vi "Barcode 2D_Setting_UI.vi"(6 "Analysis_Setting In":T2={"PreProcess"=enum."*Algorithm*", "Parameter"=""}, 8 "error in (no error)":errorcluster, 9 "ProjectName":string, 10 "ROI List IN":refnum<vi>, 11 "Vision_Image":T20(plugin-control)) -> (0 "error out":errorcluster, 1 "Cancel?":bool, 3 "Analysis_Setting":T2={"PreProcess"=enum."*Algorithm*", "Parameter"=""})   [LabVIEW 2019]
uses:
  <vilib>/vision/Instrument.llb/Demodulation Mode.ctl
  <vilib>/vision/Instrument.llb/Cell Sample Size.ctl
  <vilib>/vision/Instrument.llb/Cell Filter Mode.ctl
  <vilib>/vision/Instrument.llb/QR Code Search Options.ctl
  <vilib>/vision/Instrument.llb/Data Matrix Polarity.ctl
  <vilib>/vision/Instrument.llb/QR Code Model Type.ctl
  <vilib>/vision/Instrument.llb/QR Code Description Options.ctl
  Controls/_UI Command Cluster/Barcode 2D_UI Command Cluster.ctl
  Controls/Analysis_Type.ctl
  Controls/Analysis_Setting.ctl
  Controls/Barcode 2D/Analysis_Barcode 2D_Parameter.ctl
  <vilib>/vision/Instrument.llb/Data Matrix Search Options.ctl
  <vilib>/vision/Instrument.llb/Data Matrix Mirror.ctl
  <vilib>/vision/Instrument.llb/Cell Fill Percentage.ctl
  <vilib>/vision/Instrument.llb/ECC Type.ctl
  <vilib>/vision/Instrument.llb/Data Matrix Description Options.ctl
  <vilib>/vision/Instrument.llb/Data Matrix Advanced Options.ctl
  <vilib>/vision/Instrument.llb/Data Matrix Size Options.ctl
  Controls/V_Analysis_Type.ctl
  Ctrl/VisionProcessName.ctl
panel:
  in  "ROI":T1
  in  "Done":bool
  in  "Cancel":bool
  in  "ClampTab":T4(tab)
  in  "Suggest":bool
  in  "Barcode Type":enum16{"Data Matrix", "PDF417", "QR Code"}(ring)
  in  "Data Matrix Description Options":T5={"Aspect Ratio"=0.0, "Rows"=0, "Columns"=0, "Rectangle"=FALSE, "ECC"=-2, "Barcode Polarity"=-2, "Cell Fill Percentage"=-2, "Minimum Border Integrity %"=80.0, "Mirror Mode"=-2} {"Mirror Mode" items=["Auto-detect"=-2, "Normal"=0, "Mirrored"=1]; "ECC" items=["Auto-detect"=-2, "ECC 000"=0, "ECC 050"=50, "ECC 080"=80, "ECC 100"=100, "ECC 140"=140, "ECC 000-140"=190, "ECC 200"=200]; "Minimum Border Integrity %" format="%.2f"; "Aspect Ratio" format="%.2f"; "Cell Fill Percentage" items=["Auto-detect"=-2, "< 30%"=0, ">= 30%"=1]; "Barcode Polarity" items=["Auto-detect"=-2, "Black on White"=0, "White on Black"=1]}
  in  "Data Matrix Search Options":T10={"Rotation Mode"=enum."Unlimited", "Skip Location?"=FALSE, "Edge Threshold"=30, "Demodulation Mode"=-2, "Cell Sample Size"=-2, "Cell Filter Mode"=-2, "Skew Degrees Allowed"=5, "Maximum Iterations"=500, "Initial Search Vector Width"=5} {"Cell Filter Mode" items=["Auto-detect"=-2, "Average"=0, "Median"=1, "Central Average"=2, "High Average"=3, "Low Average"=4, "Very High Average"=5, "Very Low Average"=6, "All Filters"=8]; "Cell Sample Size" items=["Auto-detect"=-2, "1x1"=1, "2x2"=2, "3x3"=3, "4x4"=4, "5x5"=5, "6x6"=6, "7x7"=7]; "Demodulation Mode" items=["Auto-detect"=-2, "Histogram"=0, "Local Contrast"=1, "Combination"=2, "All"=3]}
  in  "Data Matrix Size Options":T14={"Data Matrix Size"={"Minimum Size"=0, "Maximum Size"=0}, "Quiet Zone Width"=10}
  in  "Advanced Options":T15[](array[typedef]) {"Value" format="%.2f"}
  in  "Search Mode":T16=enum."Single Barcode, Conservative"
  in  "QR Search Options":T17={"Rotation Mode"=enum."Unlimited", "Skip Location?"=FALSE, "Edge Threshold"=50, "Demodulation Mode"=-2, "Cell Sample Size"=-2, "Cell Filter Mode"=-2, "Skew Degrees Allowed"=5} {"Cell Filter Mode" items=["Auto-detect"=-2, "Average"=0, "Median"=1, "Central Average"=2, "High Average"=3, "Low Average"=4, "Very High Average"=5, "Very Low Average"=6, "All Filters"=8]; "Cell Sample Size" items=["Auto-detect"=-2, "1x1"=1, "2x2"=2, "3x3"=3, "4x4"=4, "5x5"=5, "6x6"=6, "7x7"=7]; "Demodulation Mode" items=["Auto-detect"=-2, "Histogram"=0, "Local Contrast"=1, "Combination"=2, "All"=3]}
  in  "QR Description Options":T18={"Matrix Size (cells)"=0, "Barcode Polarity"=0, "Mirror Mode"=0, "QR Model"=3} {"Mirror Mode" items=["Auto-detect"=-2, "Normal"=0, "Mirrored"=1]; "Matrix Size (cells)" items=["Auto-detect"=0, "11x11 - Version 1 (Micro QR Only)"=11, "13x13 - Version 2 (Micro QR Only)"=13, "15x15 - Version 3 (Micro QR Only)"=15, "17x17 - Version 4 (Micro QR Only)"=17, "21x21 - Version 1"=21, "25x25 - Version 2"=25, "29x29 - Version 3"=29, "33x33 - Version 4"=33, "37x37 - Version 5"=37, "41x41 - Version 6"=41, "45x45 - Version 7"=45, "49x49 - Version 8"=49, "53x53 - Version 9"=53, "57x57 - Version 10"=57, "61x61 - Version 11"=61, "65x65 - Version 12"=65, "69x69 - Version 13"=69, "73x73 - Version 14"=73, "77x77 - Version 15"=77, "81x81 - Version 16"=81, "85x85 - Version 17"=85, "89x89 - Version 18"=89, "93x93 - Version 19"=93, "97x97 - Version 20"=97, "101x101 - Version 21"=101, "105x105 - Version 22"=105, "109x109 - Version 23"=109, "113x113 - Version 24"=113, "117x117 - Version 25"=117, "121x121 - Version 26"=121, "125x125 - Version 27"=125, "129x129 - Version 28"=129, "133x133 - Version 29"=133, "137x137 - Version 30"=137, "141x141 - Version 31"=141, "145x145 - Version 32"=145, "149x149 - Version 33"=149, "153x153 - Version 34"=153, "157x157 - Version 35"=157, "161x161 - Version 36"=161, "165x165 - Version 37"=165, "169x169 -  Version 38"=169, "173x173 - Version 39"=173, "177x177 - Version 40"=177]; "QR Model" items=["Auto-detect", "Micro", "Model 1", "Model 2"]; "Barcode Polarity" items=["Auto-detect"=-2, "Black on White"=0, "White on Black"=1]}
  in  "QR Code Cell Size":cluster{"Minimum Size":u32, "Maximum Size":u32}={"Minimum Size"=3, "Maximum Size"=7}
  out "Barcode Result Out":string
  out "Bounding Box":cluster{"x":sgl, "y":sgl}[](array[cluster])
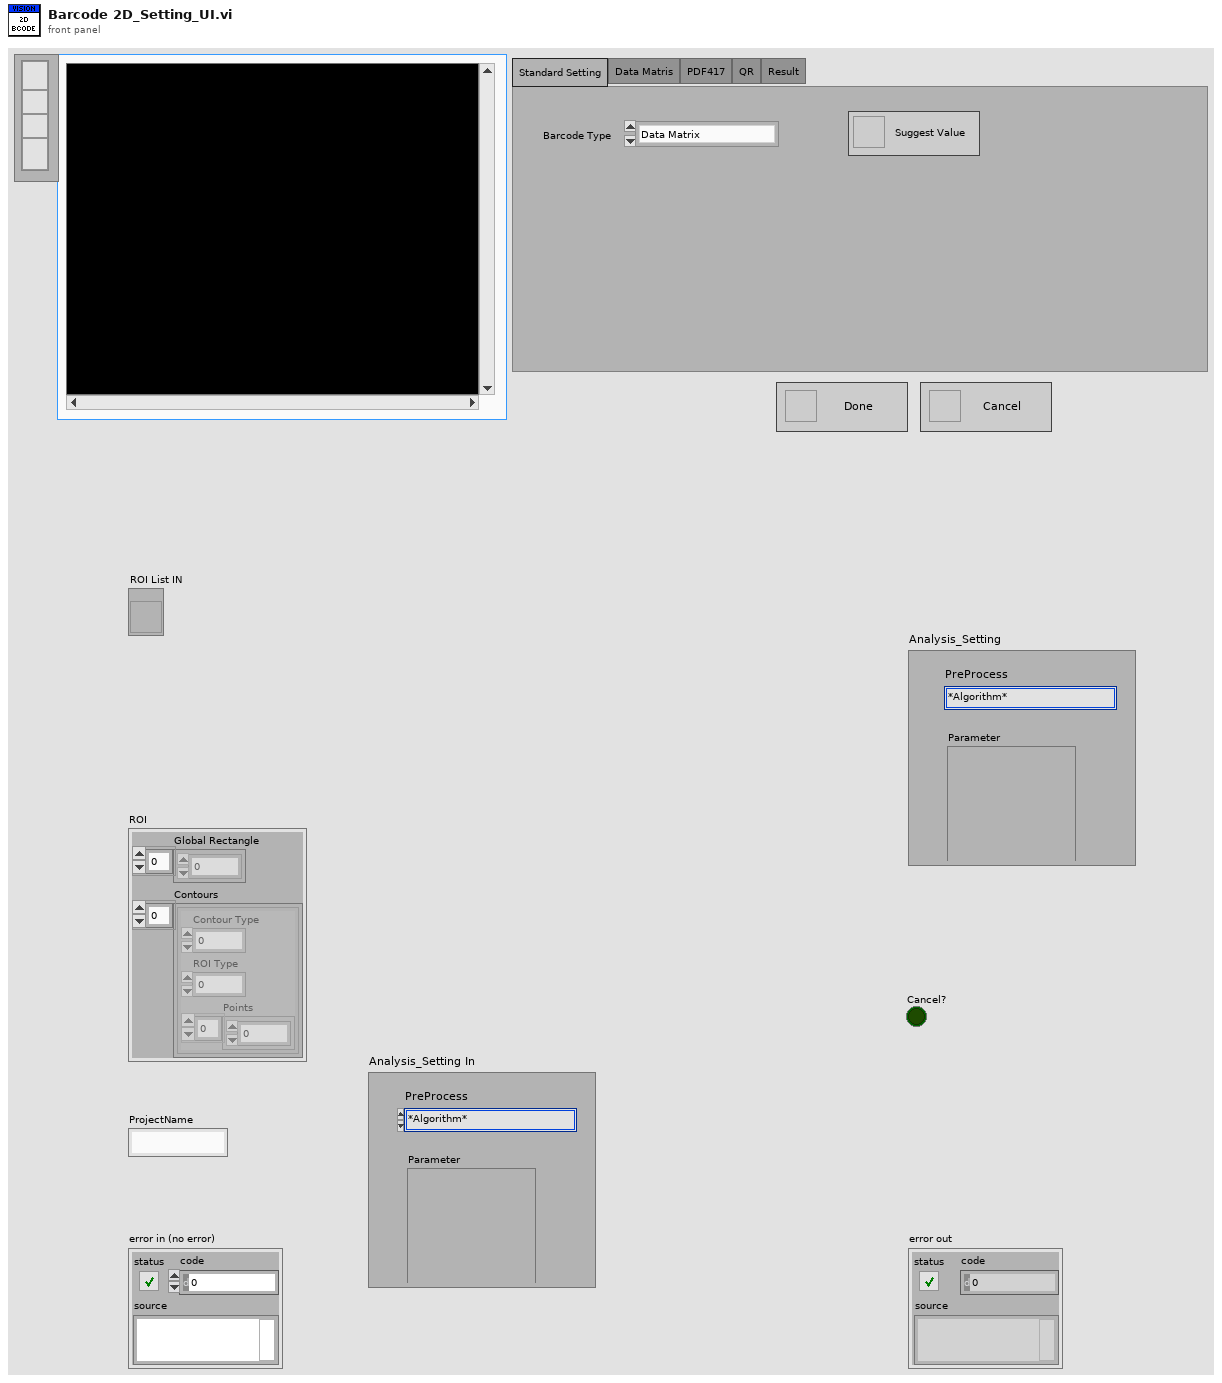
[diagram p1: front panel]
types:
  T1 = cluster{"Global Rectangle":i32[], "Contours":cluster{"Contour Type":u32, "ROI Type":u32, "Points":i32[]}[]}
  T2 = typedef "Analysis_Setting.ctl" = cluster{"PreProcess":T3, "Parameter":string}
  T3 = typedef "VisionProcessName.ctl" = enum16{"*CamParameter*", "CamAttributes", "*Preprocess*", "CG_Brightness", "C_Plane Extraction", "C_Threshold", "G_Lookup Table", "G_Threshold", "B_Image Inversion", "*Algorithm*", "CG_Histogram", "C_Color Matching", "C_Color Pattern Matching", "G_PatternMatch", "CG_Find Straight Edge", "CG_Adv. Find Straight Edge", "CG_Find Circular Edge", "G_Max Clamp", "G_Clamp (Rake)", "G_Pattern Matching"}
  T4 = enum32{"Standard Setting", "Data Matris", "PDF417", "QR", "Result"}
  T5 = typedef "Data Matrix Description Options.ctl" = cluster{"Aspect Ratio":sgl, "Rows":u32, "Columns":u32, "Rectangle":bool, "ECC":T6, "Barcode Polarity":T7, "Cell Fill Percentage":T8, "Minimum Border Integrity %":sgl, "Mirror Mode":T9}
  T6 = typedef "ECC Type.ctl" = i32
  T7 = typedef "Data Matrix Polarity.ctl" = i32
  T8 = typedef "Cell Fill Percentage.ctl" = i32
  T9 = typedef "Data Matrix Mirror.ctl" = i32
  T10 = typedef "Data Matrix Search Options.ctl" = cluster{"Rotation Mode":enum32{"Unlimited", "0 Degrees", "90 Degrees", "180 Degrees", "270 Degrees"}, "Skip Location?":bool, "Edge Threshold":u32, "Demodulation Mode":T11, "Cell Sample Size":T12, "Cell Filter Mode":T13, "Skew Degrees Allowed":u32, "Maximum Iterations":u32, "Initial Search Vector Width":u32}
  T11 = typedef "Demodulation Mode.ctl" = i32
  T12 = typedef "Cell Sample Size.ctl" = i32
  T13 = typedef "Cell Filter Mode.ctl" = i32
  T14 = typedef "Data Matrix Size Options.ctl" = cluster{"Data Matrix Size":cluster{"Minimum Size":u32, "Maximum Size":u32}, "Quiet Zone Width":u32}
  T15 = typedef "Data Matrix Advanced Options.ctl" = cluster{"Option":enum32{"Line Detection", "HighLight Filter", "Aggressive", "FNC1", "Refine Bounding Box"}, " Value":dbl}
  T16 = typedef "PDF417 Search Mode" = enum32{"Multiple Barcodes", "Single Barcode, Conservative"}
  T17 = typedef "QR Code Search Options.ctl" = cluster{"Rotation Mode":enum32{"Unlimited", "0 Degrees", "90 Degrees", "180 Degrees", "270 Degrees"}, "Skip Location?":bool, "Edge Threshold":u32, "Demodulation Mode":T11, "Cell Sample Size":T12, "Cell Filter Mode":T13, "Skew Degrees Allowed":u32}
  T18 = typedef "QR Code Description Options.ctl" = cluster{"Matrix Size (cells)":i32, "Barcode Polarity":T7, "Mirror Mode":i32, "QR Model":T19}
  T19 = typedef "QR Code Model Type.ctl" = i32
  T20 = typedef "IMAQ Image.ctl" = refnum<image>
  T21 = typedef "Barcode 2D_UI Command Cluster.ctl" = cluster{"Message":enum16{"Initialize", "InitializeUI", "Run Algorithm", "Done", "Cancel", "Exit"}, "Data":variant}
  T22 = typedef "IMAQ Line" = cluster{"Start X":i32, "Start Y":i32, "End X":i32, "End Y":i32}
  T23 = cluster{"QR Search Options":T17, "QR Description Options":T18, "QR Code Cell Size (pixels)":cluster{"Minimum Size":u32, "Maximum Size":u32}}
  T24 = cluster{"Data Matrix Description Options":T5, "Data Matrix Search Options":T10, "Data Matrix Size Options":T14, "Advanced Options":T15[]}
  T25 = typedef "Analysis_Barcode 2D_Parameter.ctl" = cluster{"ROI":cluster{"Global Rectangle":i32[], "Contours":cluster{"Contour Type":u32, "ROI Type":u32, "Points":i32[]}[]}, "Barcode Type":enum16{"Data Matrix", "PDF417", "QR Code"}, "Data Matrix Parameter":cluster{"Data Matrix Description Options":T5, "Data Matrix Search Options":T10, "Data Matrix Size Options":T14, "Advanced Options":T15[]}, "PDF147 Search Mode":T16, "QR Code Parameter":cluster{"QR Search Options":T17, "QR Description Options":T18, "QR Code Cell Size (pixels)":cluster{"Minimum Size":u32, "Maximum Size":u32}}}
  T26 = cluster{"Contour Type":u32, "ROI Type":u32, "Points":i32[]}
  T27 = enum16{"Initialize", "InitializeUI", "Run Algorithm", "Done", "Cancel", "Exit"}
  T28 = typedef "Image Type" = u32
  T29 = typedef "Analysis_Type.ctl" = u16
  T30 = typedef "Analysis_Setting.ctl" = cluster{"PreProcess":T31, "Parameter":string}
  T31 = typedef "V_Analysis_Type.ctl" = enum16{"None", "C_Color Pattern Matching", "G_PatternMatching", "G_ShapeDectect", "G_GeometricMatch", "B_Area Check"}
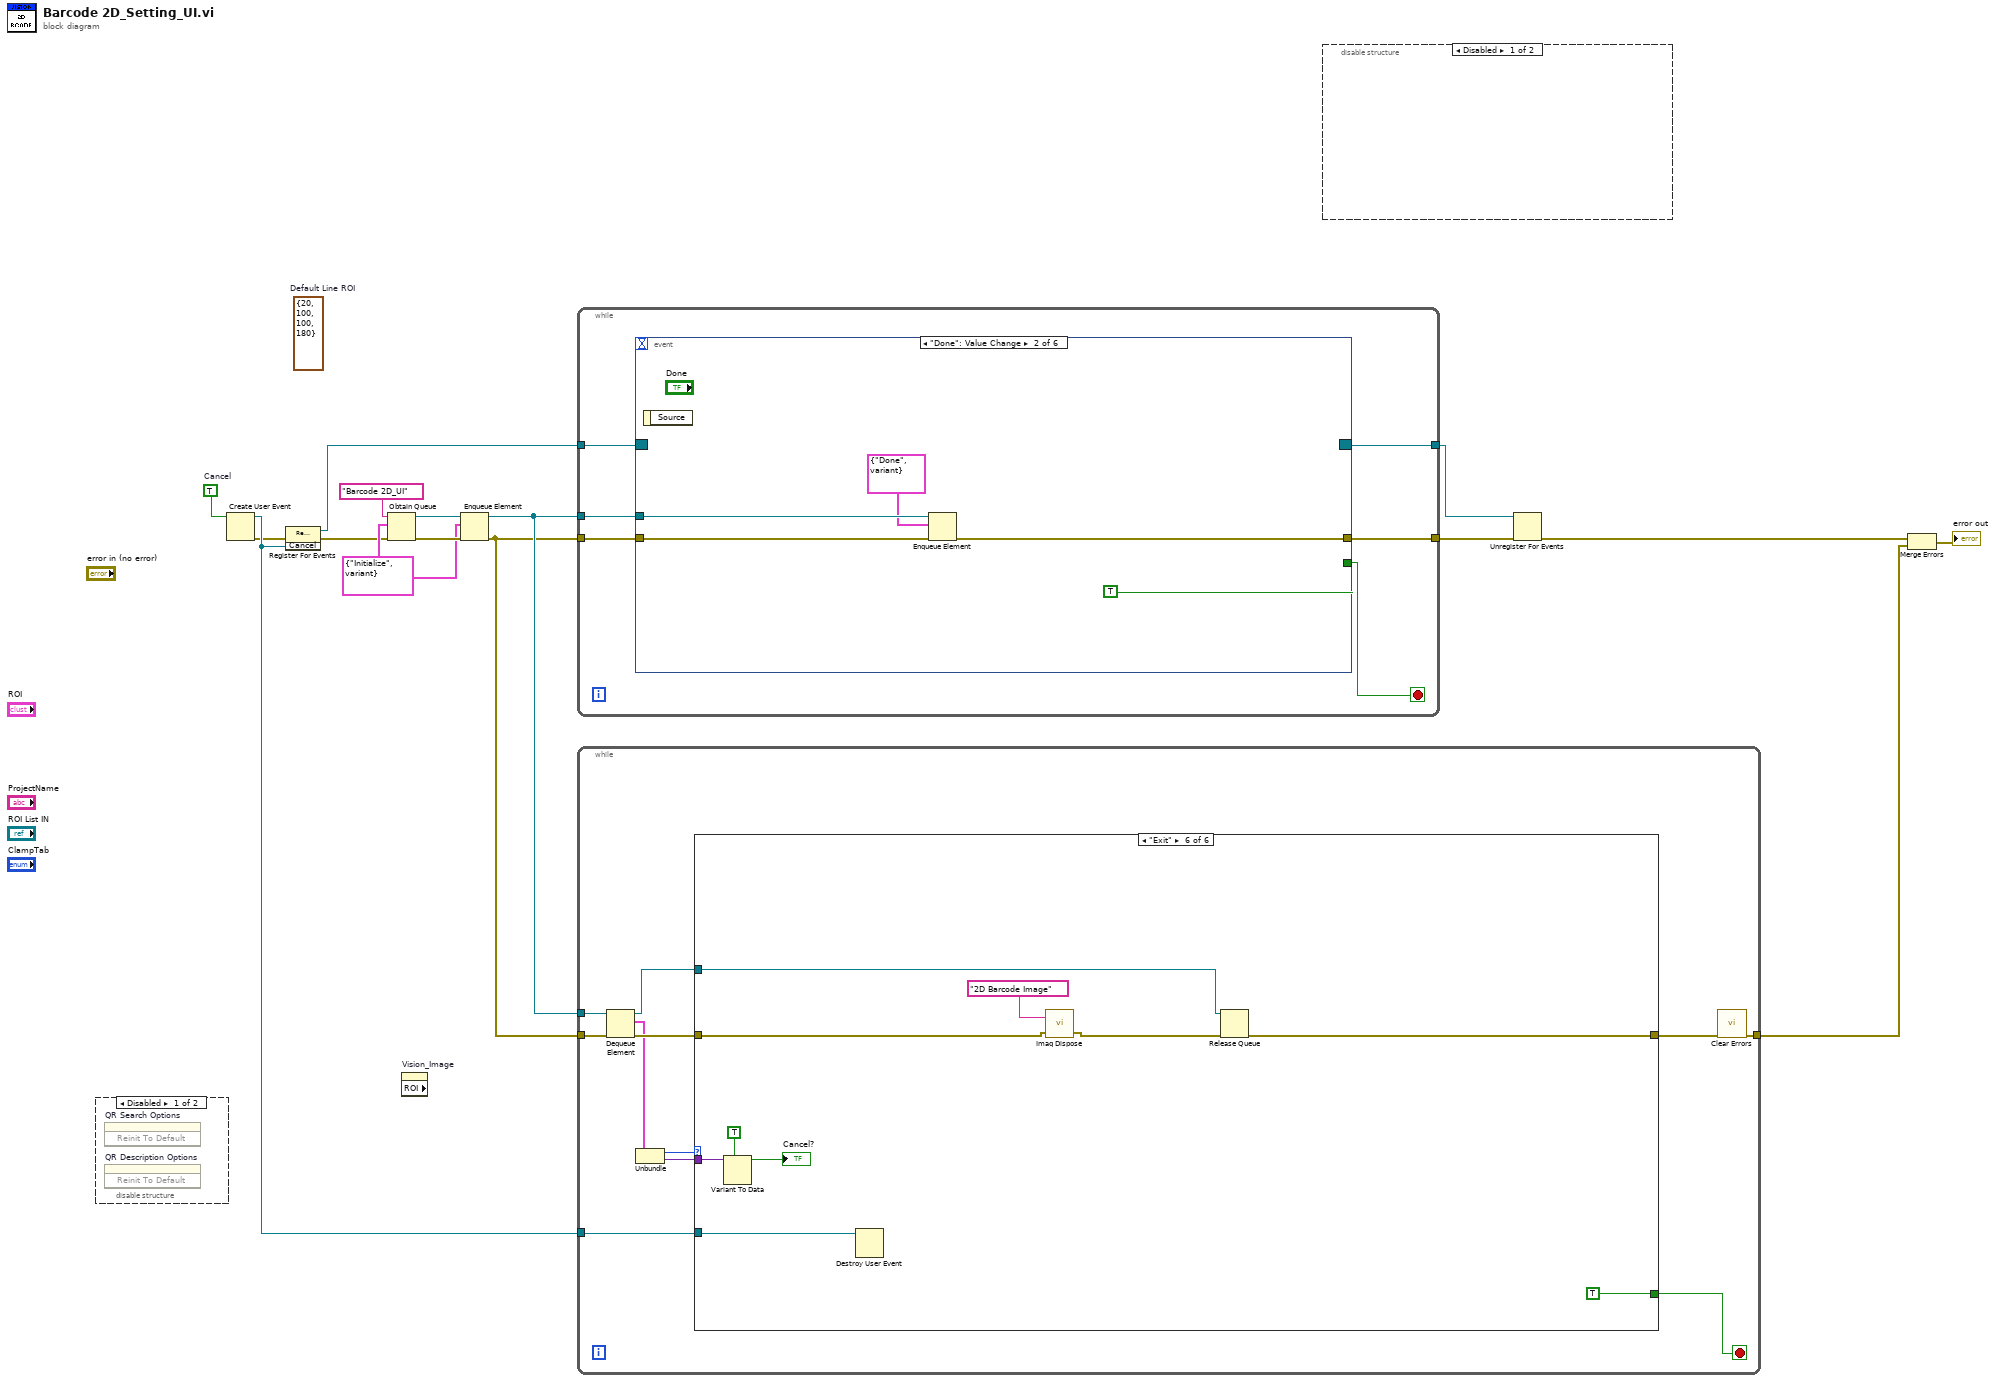
[diagram p0: block diagram]
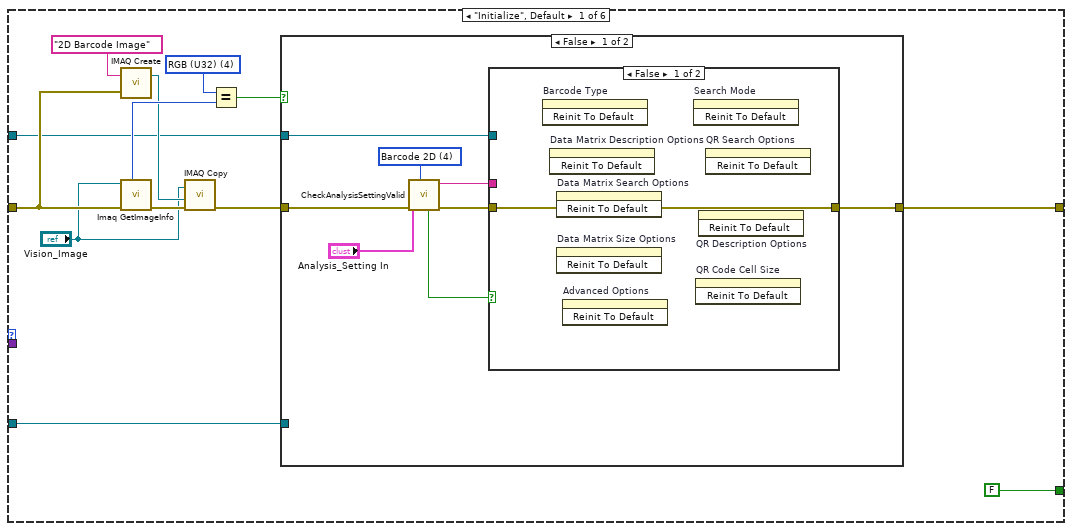
[diagram p4: hidden frame]
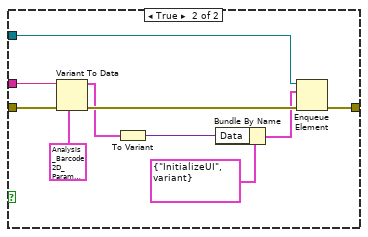
[diagram p5: hidden frame]
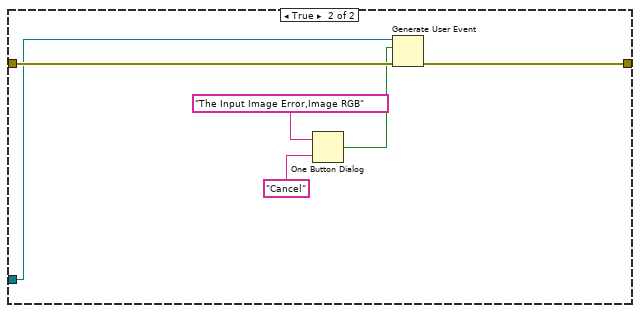
[diagram p6: hidden frame]
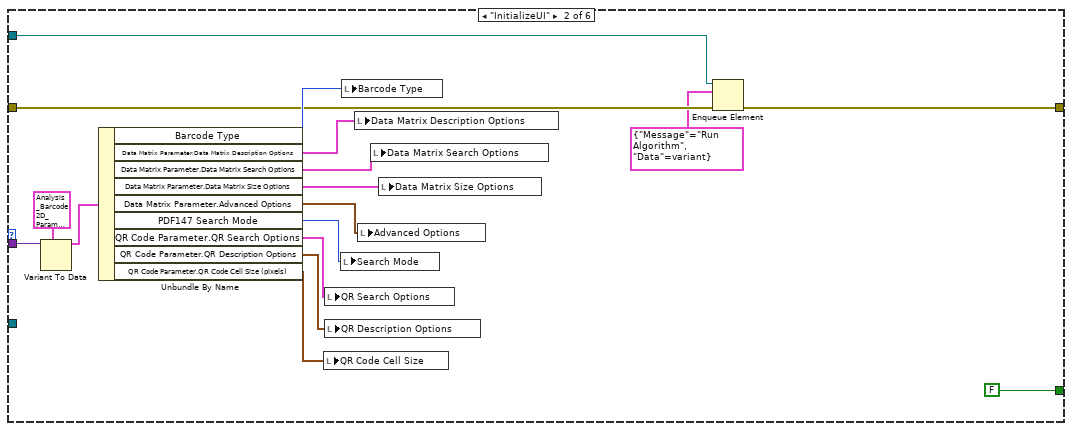
[diagram p7: hidden frame]
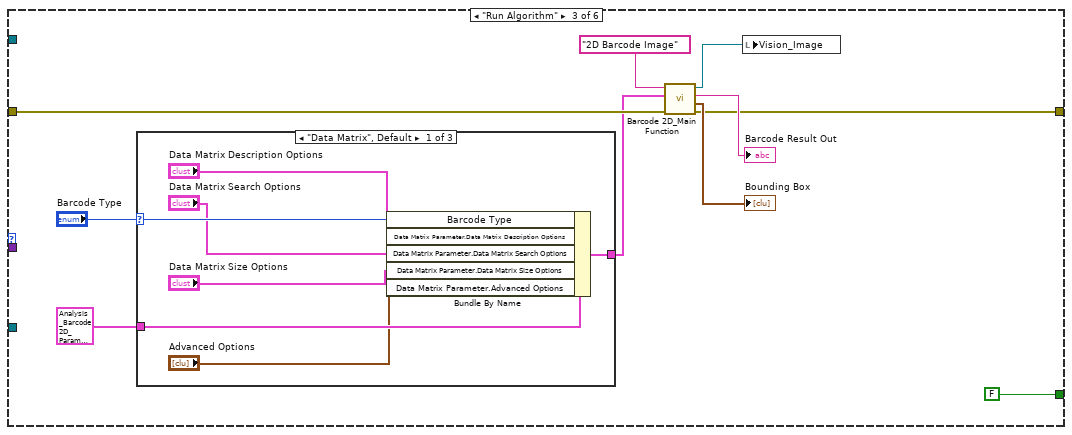
[diagram p8: hidden frame]
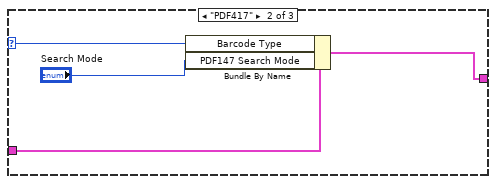
[diagram p9: hidden frame]
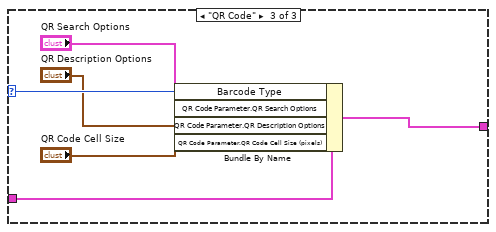
[diagram p10: hidden frame]
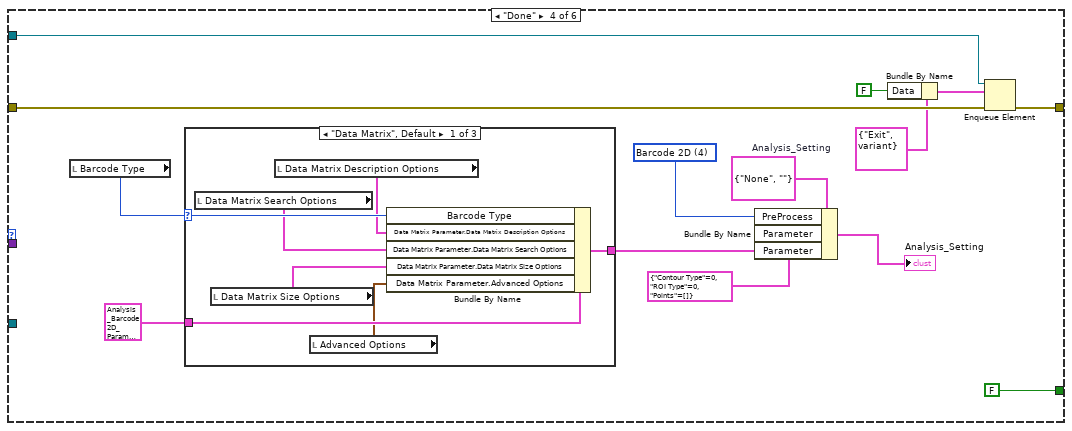
[diagram p11: hidden frame]
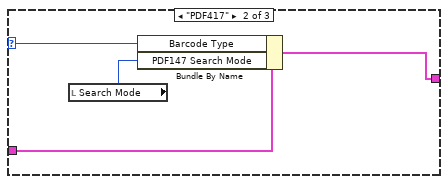
[diagram p12: hidden frame]
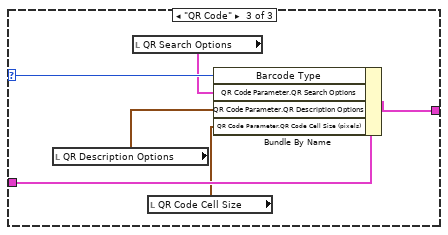
[diagram p13: hidden frame]
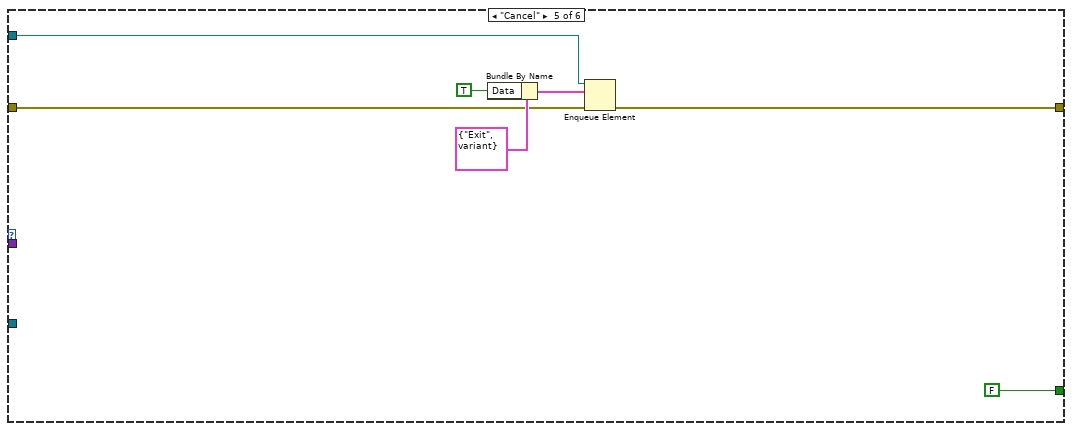
[diagram p14: hidden frame]
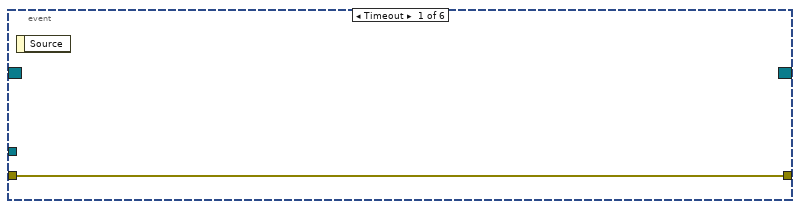
[diagram p15: hidden frame]
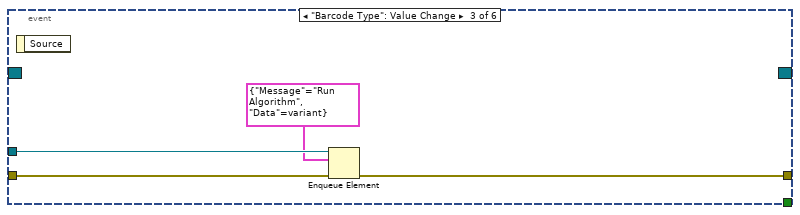
[diagram p16: hidden frame]
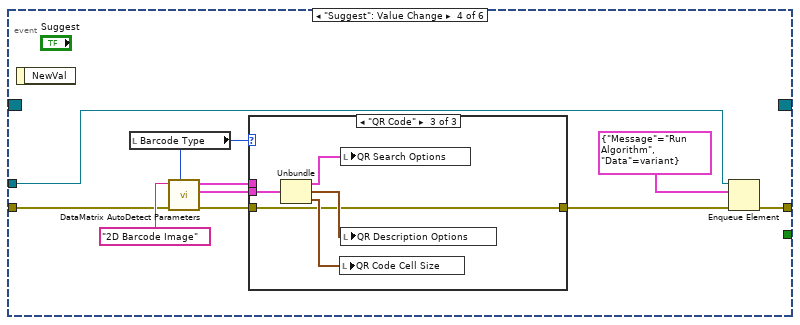
[diagram p17: hidden frame]
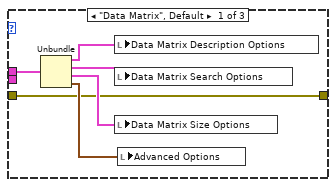
[diagram p18: hidden frame]
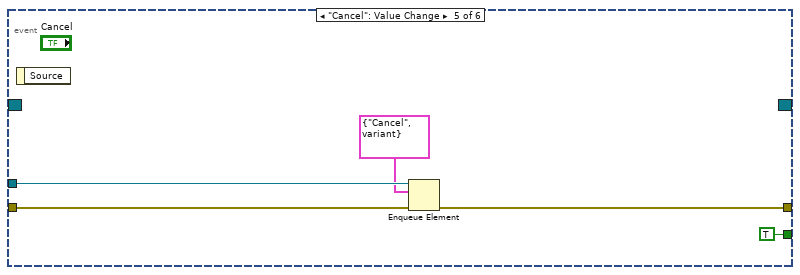
[diagram p20: hidden frame]
diagram:
  w10 = TRUE  # Cancel
  w6 = T21 {"Message"=enum."Initialize", "Data"=variant} ("Barcode 2D_UI Command")
  (unwired) T22 {"Start X"=20, "Start Y"=100, "End X"=100, "End Y"=180}  # Default Line ROI
  n1 = disable-structure shown="Disabled" {
    frame Disabled {
      n2 = invoke on="QR Search Options" class="Clust (strict)" method="Reinit To Default"() -> ()  [unwired: 3 in, 3 out]
      n3 = invoke on="QR Description Options" class="Clust (strict)" method="Reinit To Default"() -> ()  [unwired: 3 in, 3 out]
    }
    frame Enabled {
    }
  }
  n4 = Create User Event(user event datatype=w10) -> (user event=w7:refnum<user-event>, error out=w5:errorcluster)  [unwired: 1 in]
  n5 = register-events(error in=w5, w7) -> (reference out=w9:refnum<event-registration>, error out=w4:errorcluster)  [unwired: 1 in]
  n6 = Obtain Queue(name (unnamed)="Barcode 2D_UI", element data type=w6, error in (no error)=w4) -> (queue out=w16:refnum<queue>, error out=w15:errorcluster)  [unwired: 2 in, 1 out]
  n7 = property on="Vision_Image" class="ImageControl" props=["ROI"]() -> ()  [unwired: 2 in, 3 out]
  n8 = Enqueue Element(queue=w16, element=w6, error in (no error)=w15) -> (queue out=w13:refnum<queue>, error out=w12:errorcluster)  [unwired: 1 in, 1 out]
  n9 = while {
    tunnel: w13 -> [w22]
    tunnel: w12 -> [w21]
    tunnel: [w19] -> w3
    tunnel: w9 -> [w18]
    tunnel: [w17] -> w8
    stop <- w20 stop-if-true
    n10 = event shown="[1] \"Done\": Value Change" {
      selector: w18 -> [_ _ _ _ _ _]
      dyn-events: [_ _ _ _ _ _] -> w17
      timeout: _ -> [_ _ _ _ _ _]
      tunnel: w22 -> [_ w28 w32 w42 w59 w62]
      tunnel: w21 -> [w23 w27 w30 w38 w58 w61]
      tunnel: [_ TRUE _ _ TRUE TRUE] -> w20
      tunnel: [w23 w26 w31 w41 w57 _] -> w19
      event Timeout {
        n11 = event-data() -> ()  [unwired: 1 in, 1 out]
      }
      event "Done": Value Change {
        n12 = event-data() -> ()  [unwired: 1 in, 1 out]
        n13 = Enqueue Element(queue=w28, element=T21 {"Message"=enum."Done", "Data"=variant} ("Barcode 2D_UI Command Cluster"), error in (no error)=w27) -> (error out=w26:errorcluster)  [unwired: 1 in, 2 out]
      }
      event "Barcode Type": Value Change {
        n14 = event-data() -> ()  [unwired: 1 in, 1 out]
        n15 = Enqueue Element(queue=w32, element=T21 {"Message"=enum."Run Algorithm", "Data"=variant} ("Barcode 2D_UI Command Cluster"), error in (no error)=w30) -> (error out=w31:errorcluster)  [unwired: 1 in, 2 out]
      }
      event "Suggest": Value Change {
        n16 = event-data() -> ()  [unwired: 1 in, 1 out]
        n17 = local read "Barcode Type"() -> (w37:enum16{"Data Matrix", "PDF417", "QR Code"})
        n18 = call "DataMatrix AutoDetect Parameters.vi"("_Barcode Type"=w37, "error in (no error)"=w38, "Image"="2D Barcode Image") -> ("error out"=w36:errorcluster, "QR Code Auto Detect Values"=w33:T23, "Data Matrix Auto Detect Values Out"=w34:T24)  [unwired: 6 in]
        n19 = case shown="\"QR Code\"" w37 {
          tunnel: w36 -> [w43 w49 w50]
          tunnel: [w43 w49 w50] -> w35
          tunnel: w34 -> [w44 _ _]
          tunnel: w33 -> [_ _ w51]
          frame "Data Matrix", Default {
            n20 = Unbundle(w44) -> ("Data Matrix Description Options"=w48:T5, "Data Matrix Search Options"=w47:T10, "Data Matrix Size Options"=w45:T14, "Advanced Options"=w46:T15[])
            n21 = local write "Data Matrix Description Options"(w48) -> ()
            n22 = local write "Data Matrix Search Options"(w47) -> ()
            n23 = local write "Data Matrix Size Options"(w45) -> ()
            n24 = local write "Advanced Options"(w46) -> ()
          }
          frame "PDF417" {
          }
          frame "QR Code" {
            n25 = Unbundle(w51) -> ("QR Search Options"=w54:T17, "QR Description Options"=w52:T18, "QR Code Cell Size (pixels)"=w53:cluster{"Minimum Size":u32, "Maximum Size":u32})
            n26 = local write "QR Code Cell Size"(w53) -> ()
            n27 = local write "QR Search Options"(w54) -> ()
            n28 = local write "QR Description Options"(w52) -> ()
          }
        }
        n29 = Enqueue Element(queue=w42, element=T21 {"Message"=enum."Run Algorithm", "Data"=variant} ("Barcode 2D_UI Command Cluster"), error in (no error)=w35) -> (error out=w41:errorcluster)  [unwired: 1 in, 2 out]
      }
      event "Cancel": Value Change {
        n30 = event-data() -> ()  [unwired: 1 in, 1 out]
        n31 = Enqueue Element(queue=w59, element=T21 {"Message"=enum."Cancel", "Data"=variant} ("Barcode 2D_UI Command Cluster"), error in (no error)=w58) -> (error out=w57:errorcluster)  [unwired: 1 in, 2 out]
      }
      event User Event {
        n32 = event-data() -> ()  [unwired: 1 in, 1 out]
        n33 = Enqueue Element(queue=w62, element=T21 {"Message"=enum."Cancel", "Data"=variant} ("Barcode 2D_UI Command Cluster"), error in (no error)=w61) -> ()  [unwired: 1 in, 3 out]
      }
    }
  }
  n34 = while {
    tunnel: w13 -> [w74]
    tunnel: w12 -> [w73]
    tunnel: [w68] -> w1
    tunnel: w7 -> [w70]
    stop <- w65 stop-if-true
    n35 = Dequeue Element(queue=w74, error in (no error)=w73) -> (queue out=w66:refnum<queue>, element=w71:T21, error out=w72:errorcluster)  [unwired: 1 in, 1 out]
    n36 = Unbundle(w71) -> ("Message"=w67:T27, "Data"=w69:variant)
    n37 = case shown="\"Exit\"" w67 {
      tunnel: w72 -> [w82 w124 w132 w162 w189 w201]
      tunnel: [w76 w121 w133 w160 w187 w198] -> w64
      tunnel: [FALSE FALSE FALSE FALSE FALSE TRUE] -> w65
      tunnel: w70 -> [w86 _ _ _ _ w203]
      tunnel: w69 -> [_ w128 _ _ _ w196]
      tunnel: w66 -> [w77 w123 _ w161 w188 w202]
      frame "Initialize", Default {
        w84 = T28 4 items=["Grayscale (U8)", "Grayscale (I16)", "Grayscale (SGL)", "Complex (CSG)", "RGB (U32)", "HSL (U32)", "RGB (U64)", "Grayscale (U16)"] ("x")
        n38 = call "IMAQ Create"("Image Name"="2D Barcode Image", "error in (no error)"=w82) -> ("New Image"=w80:T20)  [unwired: 3 in, 1 out]
        n39 = call "Imaq GetImageInfo"("error in (no error)"=w82, "Image"="Vision_Image") -> ("error out"=w81:errorcluster, "Image Type"=w85:T28)  [unwired: 2 in, 6 out]
        n40 = call "IMAQ Copy"("error in (no error)"=w81, "Image Dst"=w80, "Image Src"="Vision_Image") -> ("error out"=w78:errorcluster)  [unwired: 3 in, 1 out]
        n41 = Equal?(x=w84, y=w85) -> (x = y?=w83:bool)
        n42 = case shown="False" w83 {
          tunnel: [w95 w111] -> w76
          tunnel: w78 -> [w94 w111]
          tunnel: w86 -> [_ w107]
          tunnel: w77 -> [w88 _]
          frame False {
            w92 = T29 4 items=["None", "PatternMatch", "Edge Detection", "Barcode 1D", "Barcode 2D", "Clamp", "Clamp MAX", "Particle", "Histogram", "Straight Edge", "Circle", "Shape Detect", "OCR", "Contour", "ColorMatch"] ("Analysis_Type")
            n43 = call "CheckAnalysisSettingValid.vi"("Analysis_Type"=w92, "error in (no error)"=w94, "ParameterIn"="Analysis_Setting In") -> ("error out"=w90:errorcluster, "ParameterOut"=w91:string, "Valid"=w89:bool)  [unwired: 6 in]
            n44 = case shown="False" w89 {
              tunnel: w90 -> [w96 w104]
              tunnel: [w96 w97] -> w95
              tunnel: w91 -> [_ w106]
              tunnel: w88 -> [_ w99]
              frame False {
                n45 = invoke on="Barcode Type" class="Enum (strict)" method="Reinit To Default"() -> ()  [unwired: 3 in, 3 out]
                n46 = invoke on="Data Matrix Description Options" class="Clust (strict)" method="Reinit To Default"() -> ()  [unwired: 3 in, 3 out]
                n47 = invoke on="Data Matrix Search Options" class="Clust (strict)" method="Reinit To Default"() -> ()  [unwired: 3 in, 3 out]
                n48 = invoke on="Data Matrix Size Options" class="Clust (strict)" method="Reinit To Default"() -> ()  [unwired: 3 in, 3 out]
                n49 = invoke on="Advanced Options" class="Arr (strict)" method="Reinit To Default"() -> ()  [unwired: 3 in, 3 out]
                n50 = invoke on="Search Mode" class="Enum (strict)" method="Reinit To Default"() -> ()  [unwired: 3 in, 3 out]
                n51 = invoke on="QR Code Cell Size" class="Clust (strict)" method="Reinit To Default"() -> ()  [unwired: 3 in, 3 out]
                n52 = invoke on="QR Description Options" class="Clust (strict)" method="Reinit To Default"() -> ()  [unwired: 3 in, 3 out]
                n53 = invoke on="QR Search Options" class="Clust (strict)" method="Reinit To Default"() -> ()  [unwired: 3 in, 3 out]
              }
              frame True {
                n54 = Variant To Data(error in=w104, type=T25 {"ROI"={"Global Rectangle"=[], "Contours"=[]}, "Barcode Type"=enum."PDF417", "Data Matrix Parameter"={"Data Matrix Description Options"={"Aspect Ratio"=0.0, "Rows"=0, "Columns"=0, "Rectangle"=FALSE, "ECC"=-2, "Barcode Polarity"=0, "Cell Fill Percentage"=-2, "Minimum Border Integrity %"=80.0, "Mirror Mode"=-2}, "Data Matrix Search Options"={"Rotation Mode"=enum."Unlimited", "Skip Location?"=FALSE, "Edge Threshold"=30, "Demodulation Mode"=-2, "Cell Sample Size"=-2, "Cell Filter Mode"=-2, "Skew Degrees Allowed"=5, "Maximum Iterations"=500, "Initial Search Vector Width"=5}, "Data Matrix Size Options"={"Data Matrix Size"={"Minimum Size"=0, "Maximum Size"=0}, "Quiet Zone Width"=10}, "Advanced Options"=[]}, "PDF147 Search Mode"=enum."Multiple Barcodes", "QR Code Parameter"={"QR Search Options"={"Rotation Mode"=enum."Unlimited", "Skip Location?"=FALSE, "Edge Threshold"=30, "Demodulation Mode"=-2, "Cell Sample Size"=-2, "Cell Filter Mode"=-2, "Skew Degrees Allowed"=5}, "QR Description Options"={"Matrix Size (cells)"=0, "Barcode Polarity"=-2, "Mirror Mode"=-2, "QR Model"=0}, "QR Code Cell Size (pixels)"={"Minimum Size"=3, "Maximum Size"=7}}} ("Analysis_Barcode 2D_Parameter"), Variant=w106) -> (data=w101:T25, error out=w103:errorcluster)
                n55 = To Variant(anything=w101) -> (Variant=w100:variant)
                n56 = Bundle By Name(cluster=T21 {"Message"=enum."InitializeUI", "Data"=variant} ("Barcode 2D_UI Command"), "Data"=w100) -> (w98:T21)
                n57 = Enqueue Element(queue=w99, element=w98, error in (no error)=w103) -> (error out=w97:errorcluster)  [unwired: 1 in, 2 out]
              }
            }
          }
          frame True {
            n58 = One Button Dialog(message="The Input Image Error,Image RGB", button name ("OK")="Cancel") -> (true=w108:bool)
            n59 = Generate User Event(user event=w107, event data cluster=w108) -> ()  [unwired: 2 in, 2 out]
          }
        }
      }
      frame "InitializeUI" {
        n60 = Variant To Data(type=T25 {"ROI"={"Global Rectangle"=[], "Contours"=[]}, "Barcode Type"=enum."PDF417", "Data Matrix Parameter"={"Data Matrix Description Options"={"Aspect Ratio"=0.0, "Rows"=0, "Columns"=0, "Rectangle"=FALSE, "ECC"=-2, "Barcode Polarity"=0, "Cell Fill Percentage"=-2, "Minimum Border Integrity %"=80.0, "Mirror Mode"=-2}, "Data Matrix Search Options"={"Rotation Mode"=enum."Unlimited", "Skip Location?"=FALSE, "Edge Threshold"=30, "Demodulation Mode"=-2, "Cell Sample Size"=-2, "Cell Filter Mode"=-2, "Skew Degrees Allowed"=5, "Maximum Iterations"=500, "Initial Search Vector Width"=5}, "Data Matrix Size Options"={"Data Matrix Size"={"Minimum Size"=0, "Maximum Size"=0}, "Quiet Zone Width"=10}, "Advanced Options"=[]}, "PDF147 Search Mode"=enum."Multiple Barcodes", "QR Code Parameter"={"QR Search Options"={"Rotation Mode"=enum."Unlimited", "Skip Location?"=FALSE, "Edge Threshold"=30, "Demodulation Mode"=-2, "Cell Sample Size"=-2, "Cell Filter Mode"=-2, "Skew Degrees Allowed"=5}, "QR Description Options"={"Matrix Size (cells)"=0, "Barcode Polarity"=-2, "Mirror Mode"=-2, "QR Model"=0}, "QR Code Cell Size (pixels)"={"Minimum Size"=3, "Maximum Size"=7}}} ("Analysis_Barcode 2D_Parameter"), Variant=w128) -> (data=w126:T25)  [unwired: 1 in, 1 out]
        n61 = Unbundle By Name(w126) -> ("Barcode Type"=w125:enum16{"Data Matrix", "PDF417", "QR Code"}, "Data Matrix Parameter.Data Matrix Description Options"=w120:T5, "Data Matrix Parameter.Data Matrix Search Options"=w119:T10, "Data Matrix Parameter.Data Matrix Size Options"=w118:T14, "Data Matrix Parameter.Advanced Options"=w117:T15[], "PDF147 Search Mode"=w113:T16, "QR Code Parameter.QR Search Options"=w115:T17, "QR Code Parameter.QR Description Options"=w114:T18, "QR Code Parameter.QR Code Cell Size (pixels)"=w116:cluster{"Minimum Size":u32, "Maximum Size":u32})
        n62 = local write "QR Code Cell Size"(w116) -> ()
        n63 = local write "QR Search Options"(w115) -> ()
        n64 = local write "QR Description Options"(w114) -> ()
        n65 = local write "Search Mode"(w113) -> ()
        n66 = local write "Barcode Type"(w125) -> ()
        n67 = local write "Data Matrix Description Options"(w120) -> ()
        n68 = local write "Advanced Options"(w117) -> ()
        n69 = local write "Data Matrix Search Options"(w119) -> ()
        n70 = local write "Data Matrix Size Options"(w118) -> ()
        n71 = Enqueue Element(queue=w123, element=T21 {"Message"=enum."Run Algorithm", "Data"=variant} ("Barcode 2D_UI Command"), error in (no error)=w124) -> (error out=w121:errorcluster)  [unwired: 1 in, 2 out]
      }
      frame "Run Algorithm" {
        n72 = case shown="\"Data Matrix\", Default" "Barcode Type" {
          selector: "Barcode Type" -> [w145 w149 w155]
          tunnel: T25 {"ROI"={"Global Rectangle"=[], "Contours"=[]}, "Barcode Type"=enum."PDF417", "Data Matrix Parameter"={"Data Matrix Description Options"={"Aspect Ratio"=0.0, "Rows"=0, "Columns"=0, "Rectangle"=FALSE, "ECC"=-2, "Barcode Polarity"=0, "Cell Fill Percentage"=-2, "Minimum Border Integrity %"=80.0, "Mirror Mode"=-2}, "Data Matrix Search Options"={"Rotation Mode"=enum."Unlimited", "Skip Location?"=FALSE, "Edge Threshold"=30, "Demodulation Mode"=-2, "Cell Sample Size"=-2, "Cell Filter Mode"=-2, "Skew Degrees Allowed"=5, "Maximum Iterations"=500, "Initial Search Vector Width"=5}, "Data Matrix Size Options"={"Data Matrix Size"={"Minimum Size"=0, "Maximum Size"=0}, "Quiet Zone Width"=10}, "Advanced Options"=[]}, "PDF147 Search Mode"=enum."Multiple Barcodes", "QR Code Parameter"={"QR Search Options"={"Rotation Mode"=enum."Unlimited", "Skip Location?"=FALSE, "Edge Threshold"=30, "Demodulation Mode"=-2, "Cell Sample Size"=-2, "Cell Filter Mode"=-2, "Skew Degrees Allowed"=5}, "QR Description Options"={"Matrix Size (cells)"=0, "Barcode Polarity"=-2, "Mirror Mode"=-2, "QR Model"=0}, "QR Code Cell Size (pixels)"={"Minimum Size"=3, "Maximum Size"=7}}} ("Analysis_Barcode 2D_Parameter") -> [w144 w148 w154]
          tunnel: [w143 w147 w153] -> w131
          frame "Data Matrix", Default {
            n73 = Bundle By Name(cluster=w144, "Barcode Type"=w145, "Data Matrix Parameter.Data Matrix Description Options"="Data Matrix Description Options", "Data Matrix Parameter.Data Matrix Search Options"="Data Matrix Search Options", "Data Matrix Parameter.Data Matrix Size Options"="Data Matrix Size Options", "Data Matrix Parameter.Advanced Options"="Advanced Options") -> (w143:T25)
          }
          frame "PDF417" {
            n74 = Bundle By Name(cluster=w148, "Barcode Type"=w149, "PDF147 Search Mode"="Search Mode") -> (w147:T25)
          }
          frame "QR Code" {
            n75 = Bundle By Name(cluster=w154, "Barcode Type"=w155, "QR Code Parameter.QR Search Options"="QR Search Options", "QR Code Parameter.QR Description Options"="QR Description Options", "QR Code Parameter.QR Code Cell Size (pixels)"="QR Code Cell Size") -> (w153:T25)
          }
        }
        n76 = call "Barcode 2D_Main Function.vi"("error in (no error)"=w132, "2D Barcode Parameter in"=w131, "Image In"="2D Barcode Image") -> ("error out"=w133:errorcluster, "Bounding Box"=→"Bounding Box":cluster{"x":sgl, "y":sgl}[], "Data"=→"Barcode Result Out":string, "Image Out"=w134:T20)  [unwired: 5 in]
        n77 = local write "Vision_Image"(w134) -> ()
      }
      frame "Done" {
        w168 = T29 4 items=["None", "PatternMatch", "Edge Detection", "Barcode 1D", "Barcode 2D", "Clamp", "Clamp MAX", "Particle", "Histogram", "Straight Edge", "Circle", "Shape Detect", "OCR", "Contour", "ColorMatch"] ("Analysis_Type")
        w169 = T30 {"PreProcess"=enum."None", "Parameter"=""}  # Analysis_Setting
        n78 = local read "Barcode Type"() -> (w165:enum16{"Data Matrix", "PDF417", "QR Code"})
        n79 = case shown="\"Data Matrix\", Default" w165 {
          selector: w165 -> [w176 w180 w186]
          tunnel: T25 {"ROI"={"Global Rectangle"=[], "Contours"=[]}, "Barcode Type"=enum."PDF417", "Data Matrix Parameter"={"Data Matrix Description Options"={"Aspect Ratio"=0.0, "Rows"=0, "Columns"=0, "Rectangle"=FALSE, "ECC"=-2, "Barcode Polarity"=0, "Cell Fill Percentage"=-2, "Minimum Border Integrity %"=80.0, "Mirror Mode"=-2}, "Data Matrix Search Options"={"Rotation Mode"=enum."Unlimited", "Skip Location?"=FALSE, "Edge Threshold"=30, "Demodulation Mode"=-2, "Cell Sample Size"=-2, "Cell Filter Mode"=-2, "Skew Degrees Allowed"=5, "Maximum Iterations"=500, "Initial Search Vector Width"=5}, "Data Matrix Size Options"={"Data Matrix Size"={"Minimum Size"=0, "Maximum Size"=0}, "Quiet Zone Width"=10}, "Advanced Options"=[]}, "PDF147 Search Mode"=enum."Multiple Barcodes", "QR Code Parameter"={"QR Search Options"={"Rotation Mode"=enum."Unlimited", "Skip Location?"=FALSE, "Edge Threshold"=30, "Demodulation Mode"=-2, "Cell Sample Size"=-2, "Cell Filter Mode"=-2, "Skew Degrees Allowed"=5}, "QR Description Options"={"Matrix Size (cells)"=0, "Barcode Polarity"=-2, "Mirror Mode"=-2, "QR Model"=0}, "QR Code Cell Size (pixels)"={"Minimum Size"=3, "Maximum Size"=7}}} ("Analysis_Barcode 2D_Parameter") -> [w175 w179 w185]
          tunnel: [w174 w178 w184] -> w163
          frame "Data Matrix", Default {
            n80 = local read "Data Matrix Search Options"() -> (w170:T10)
            n81 = local read "Data Matrix Size Options"() -> (w171:T14)
            n82 = local read "Data Matrix Description Options"() -> (w173:T5)
            n83 = local read "Advanced Options"() -> (w172:T15[])
            n84 = Bundle By Name(cluster=w175, "Barcode Type"=w176, "Data Matrix Parameter.Data Matrix Description Options"=w173, "Data Matrix Parameter.Data Matrix Search Options"=w170, "Data Matrix Parameter.Data Matrix Size Options"=w171, "Data Matrix Parameter.Advanced Options"=w172) -> (w174:T25)
          }
          frame "PDF417" {
            n85 = local read "Search Mode"() -> (w177:T16)
            n86 = Bundle By Name(cluster=w179, "Barcode Type"=w180, "PDF147 Search Mode"=w177) -> (w178:T25)
          }
          frame "QR Code" {
            n87 = local read "QR Description Options"() -> (w182:T18)
            n88 = local read "QR Search Options"() -> (w183:T17)
            n89 = local read "QR Code Cell Size"() -> (w181:cluster{"Minimum Size":u32, "Maximum Size":u32})
            n90 = Bundle By Name(cluster=w185, "Barcode Type"=w186, "QR Code Parameter.QR Search Options"=w183, "QR Code Parameter.QR Description Options"=w182, "QR Code Parameter.QR Code Cell Size (pixels)"=w181) -> (w184:T25)
          }
        }
        n91 = Bundle By Name(cluster=w169, "PreProcess"=w168, "Parameter"=T26 {"Contour Type"=0, "ROI Type"=0, "Points"=[]} ("RegionContour"), "Parameter"=w163) -> (→"Analysis_Setting":T30)
        n92 = Bundle By Name(cluster=T21 {"Message"=enum."Exit", "Data"=variant} ("Barcode 2D_UI Command"), "Data"=FALSE) -> (w158:T21)
        n93 = Enqueue Element(queue=w161, element=w158, error in (no error)=w162) -> (error out=w160:errorcluster)  [unwired: 1 in, 2 out]
      }
      frame "Cancel" {
        n94 = Bundle By Name(cluster=T21 {"Message"=enum."Exit", "Data"=variant} ("Barcode 2D_UI Command"), "Data"=TRUE) -> (w191:T21)
        n95 = Enqueue Element(queue=w188, element=w191, error in (no error)=w189) -> (error out=w187:errorcluster)  [unwired: 1 in, 2 out]
      }
      frame "Exit" {
        n96 = Variant To Data(type=TRUE, Variant=w196) -> (data=→"Cancel?":bool)  [unwired: 1 in, 1 out]
        n97 = Destroy User Event(user event=w203) -> ()  [unwired: 1 in, 1 out]
        n98 = call "Imaq Dispose"("Image"="2D Barcode Image", "error in (no error)"=w201) -> ("error out"=w200:errorcluster)  [unwired: 4 in]
        n99 = Release Queue(queue=w202, error in (no error)=w200) -> (error out=w198:errorcluster)  [unwired: 1 in, 2 out]
      }
    }
    n100 = call <vilib>:"Clear Errors.vi"("error in (no error)"=w64) -> ("error out"=w68:errorcluster)  [unwired: 5 in, 1 out]
  }
  n101 = disable-structure shown="Disabled" {
    frame Disabled {
    }
    frame Enabled {
    }
  }
  n102 = Unregister For Events(event registration refnum=w8, error in=w3) -> (error out=w2:errorcluster)
  n103 = Merge Errors(w2, w1) -> (→"error out":errorcluster)
